vi "createIdStr.vi"(8 "error in (no error)":errorcluster, 10 "id":T1=1, 11 "CoolerSerialCommand in":refnum<class "CoolerSerialCommand.lvclass">) -> (0 "error out":errorcluster, 2 "idStr":string, 3 "CoolerSerialCommand out":refnum<class "CoolerSerialCommand.lvclass">)   [LabVIEW 2016, in "CoolerSerialCommand.lvclass"]
uses:
  CoolerSerialCommand.lvclass
  typedefs/CoolerId.ctl
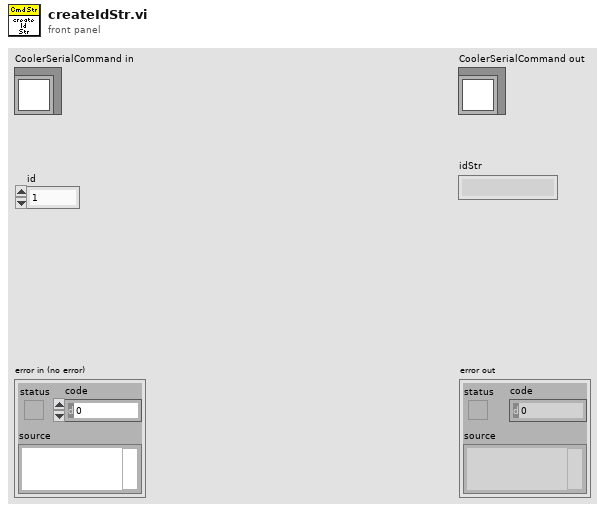
[diagram p1: front panel]
types:
  T1 = typedef "CoolerId.ctl" = u16
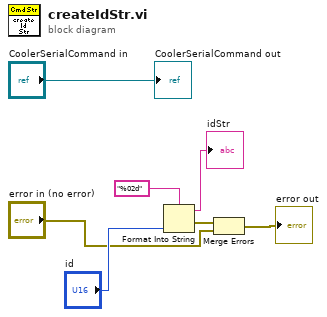
[diagram p0: block diagram]
diagram:
  n1 = Format Into String(format string="%02d", "id") -> (resulting string=→"idStr":string, error out=w2:errorcluster)  [unwired: 2 in]
  n2 = Merge Errors(w2, "error in (no error)") -> (→"error out":errorcluster)
  "CoolerSerialCommand out" <- "CoolerSerialCommand in"
